vi "Overall_system_A1-125khz.vi"() -> ()   [LabVIEW 2019]
doc: "This VI is th overall VI that can read the weight, rfid and camera (and save the data into a csv file). When certain threshold are met it can also send a telegram message at the end."
uses:
  dependencies/notification/Telegram-Bot-master (1)/Telegram-Bot-master/Telegram/Methods/TypeDefs/SendMessageType.ctl
panel:
  out "Rfid":string
  in  "RFID VISA resource name 2":refnum<visa-resource-name>="COM1"
  in  "start condition (debug)":bool
  out "Weight":string
  in  "delay before read (ms)":u32=500
  in  "Weight VISA resource name":refnum<visa-resource-name>="COM1"
  in  "Start camera (debug)":bool
  out "Health Monitoring in Progress":bool
  in  "Bird is underfeeding (debug)":bool
  out "Current image":T1(plugin-control)
  in  "Camera Name":refnum<k21>="cam0" caption="IMAQdx Session"
  # "Intelligent Health Monitoring System"
  # "grams"
  # "Weight detection settings:"
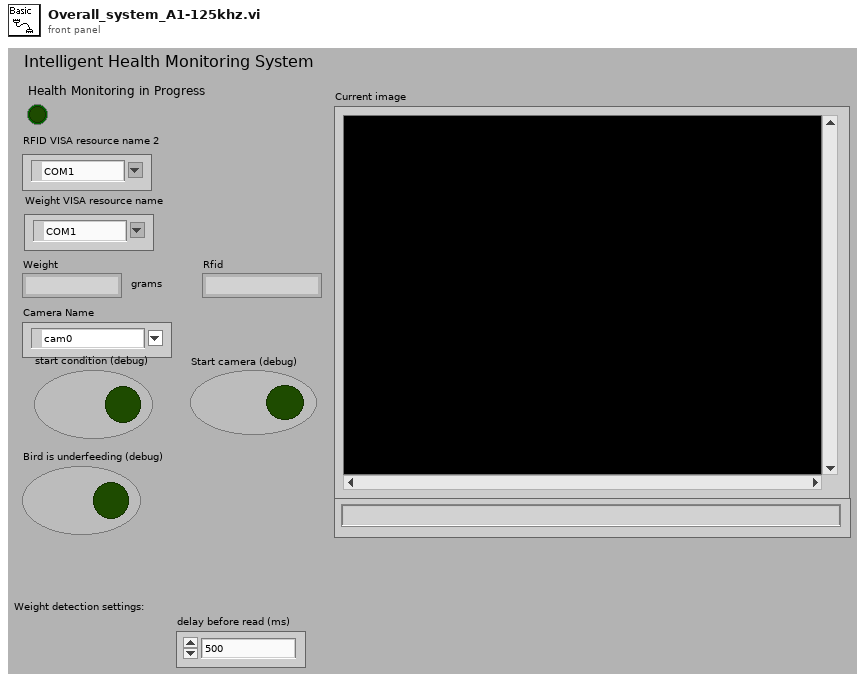
[diagram p1: front panel]
types:
  T1 = typedef "IMAQ Image.ctl" = refnum<image>
  T2 = typedef "SendMessageType.ctl" = enum16{"Text", "ReplyKeyboardMarkup", "ReplyKeyboardRemove"}
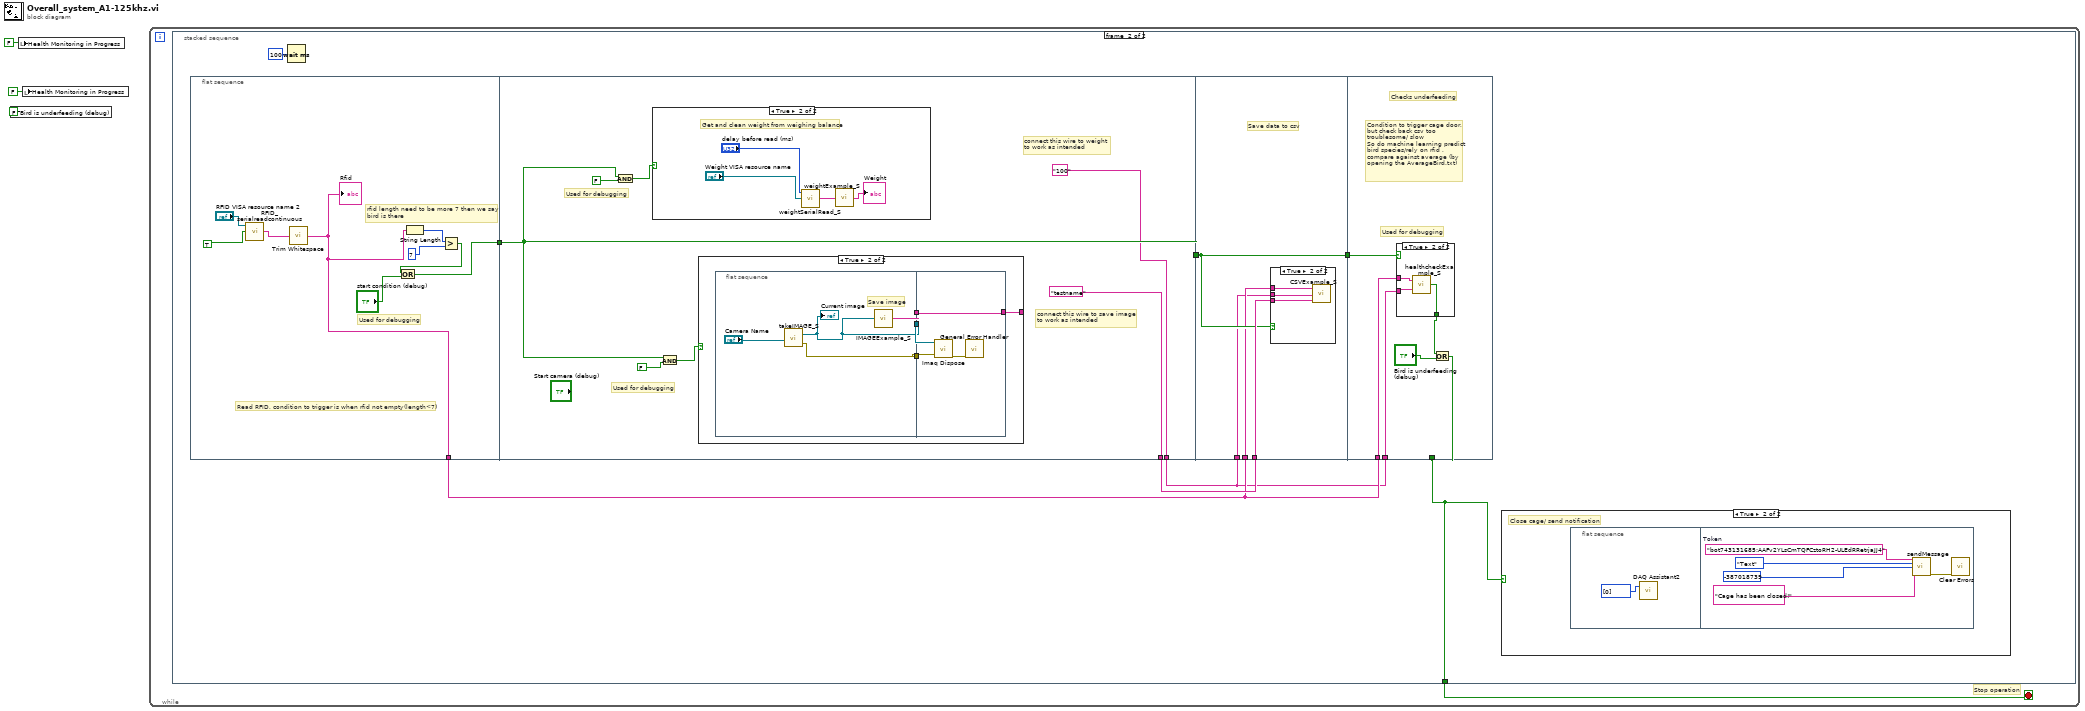
[diagram p0: block diagram]
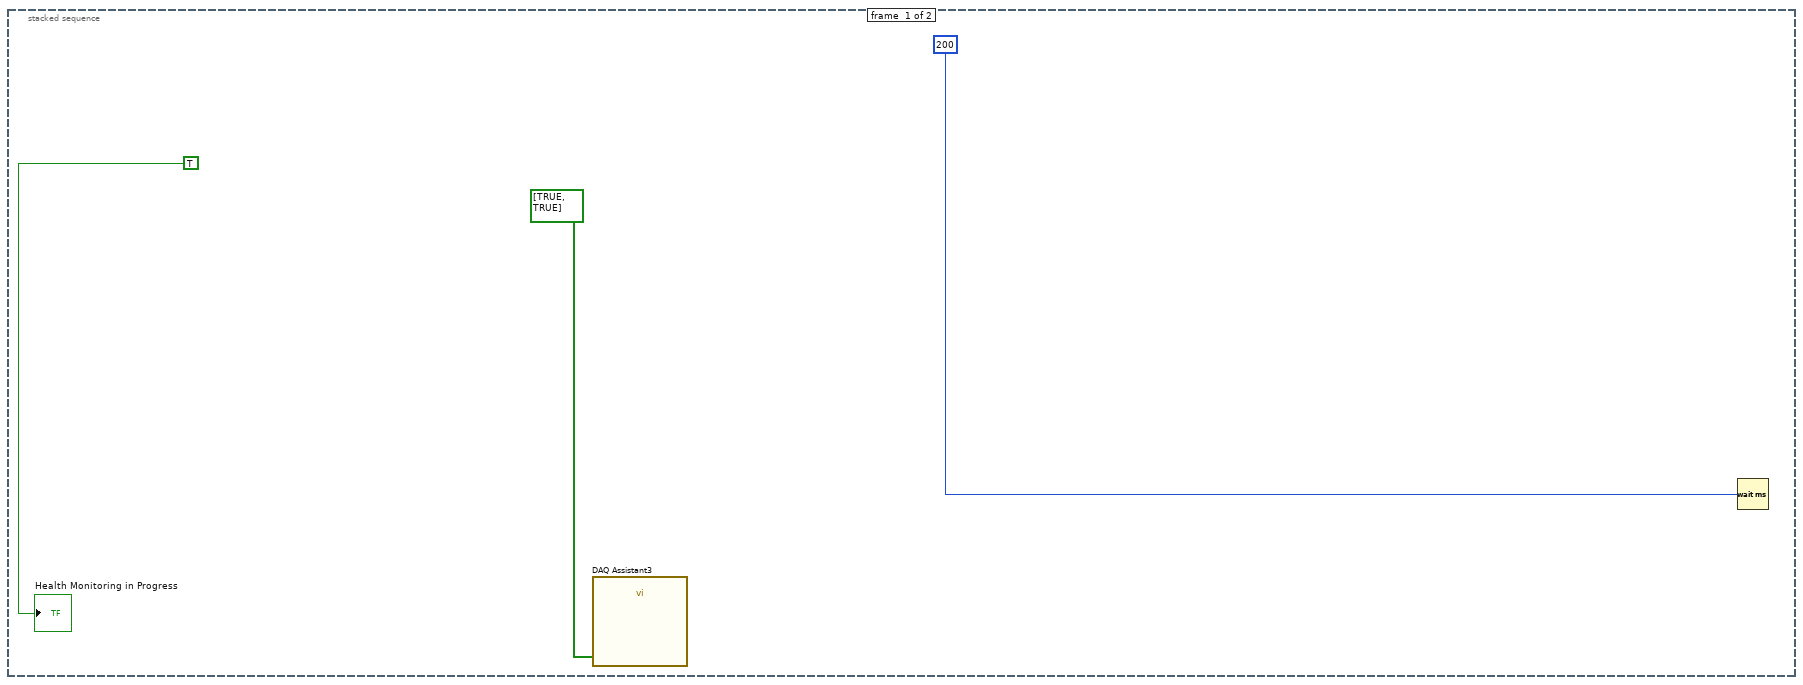
[diagram p2: hidden frame]
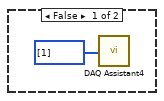
[diagram p4: hidden frame]
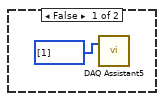
[diagram p7: hidden frame]
diagram:
  n1 = local write "Bird is underfeeding (debug)"(FALSE ("Bird is underfeeding")) -> ()
  n2 = local write "Health Monitoring in Progress"(FALSE ("Health Monitoring in Progress")) -> ()
  n3 = local write "Health Monitoring in Progress"(FALSE ("Health Monitoring in Progress")) -> ()
  n4 = while {
    stop <- w4 stop-if-true
    # "Stop operation"
    n5 = stacked-sequence {
      tunnel: [_ w14] -> w4
      frame #0 {
        n6 = call "DAQ Assistant3"("data"=bool[] [TRUE, TRUE]) -> ()  [unwired: 17 in, 2 out]
        n7 = Wait (ms)(milliseconds to wait=u32 200) -> ()  [unwired: 1 out]
        "Health Monitoring in Progress" <- TRUE ("Health Monitoring in Progress")
      }
      frame #1 {
        n8 = flat-sequence {
          tunnel: [w19] -> w9
          tunnel: [w23] -> w13
          tunnel: ["100"] -> w8
          tunnel: ["testname"] -> w10
          tunnel: w13 -> [w27]
          tunnel: [w27] -> w12
          tunnel: w12 -> [w51]
          tunnel: [w51] -> w11
          tunnel: w10 -> [w52]
          tunnel: w9 -> [w50]
          tunnel: w8 -> [w49]
          tunnel: [w58] -> w14
          tunnel: w9 -> [w57]
          tunnel: w11 -> [w61]
          tunnel: w8 -> [w56]
          frame #0 {
            # "Used for debugging"
            # "rfid length need to be more 7 then we say \nbird is there"
            # "Read RFID, condition to trigger is when rfid not empty(length<7)"
            n9 = call "RFID_serialreadcontinuous.vi"("Read 2"=TRUE, "VISA resource name"="RFID VISA resource name 2") -> ("Response 2"=w18:string)  [unwired: 1 in]
            n10 = call <vilib>:"Trim Whitespace.vi"("string"=w18) -> ("trimmed string"=w19:string)  [unwired: 1 in]
            "Rfid" <- w19
            n11 = String Length(string=w19) -> (length=w22:i32)
            n12 = Greater?(x=w22, y=7) -> (0:w20:bool)
            n13 = Or(x=w20, y="start condition (debug)") -> (x .or. y?=w23:bool)
          }
          frame #1 {
            # "connect this wire to save image \nto work as intended"
            # "connect this wire to weight \nto work as intended"
            # "Used for debugging"
            # "Used for debugging"
            n14 = And(x=w27, y=FALSE) -> (x .and. y?=w26:bool)
            n15 = case shown="True" w26 {
              frame False {
                n16 = call "DAQ Assistant4"("data"=u32[] [1]) -> ()  [unwired: 17 in, 2 out]
              }
              frame True {
                # "Get and clean weight from weighing balance"
                n17 = call "weightSerialRead_S.vi"("Weight VISA resource name"="Weight VISA resource name", "delay before read (ms)"="delay before read (ms)") -> ("String"=w48:string)  [unwired: 1 in]
                n18 = call "weightExample_S.vi"("weight"=w48) -> ("String"=→"Weight":string)
              }
            }
            n19 = And(x=w27, y=FALSE) -> (x .and. y?=w30:bool)
            n20 = case shown="True" w30 {
              tunnel: [_ w33] -> _
              frame False {
              }
              frame True {
                n21 = flat-sequence {
                  tunnel: [w37] -> w35
                  tunnel: [w36] -> w34
                  tunnel: [w39] -> w32
                  tunnel: w35 -> [w43]
                  tunnel: w34 -> [w41]
                  tunnel: [w40] -> w33
                  tunnel: w32 -> [w40]
                  frame #0 {
                    # "Save image"
                    n22 = call "takeIMAGE_S.vi"("Camera Name"="Camera Name") -> ("Current image"=w36:T1, "error in (no error)"=w37:errorcluster)
                    "Current image" <- w36
                    n23 = call "IMAGEExample_S.vi"("Image"=w36) -> ("String"=w39:string)
                  }
                  frame #1 {
                    n24 = call "Imaq Dispose"("Image"=w41, "error in (no error)"=w43) -> ("error out"=w42:errorcluster)  [unwired: 4 in]
                    n25 = call <vilib>:"General Error Handler.vi"("error in (no error)"=w42) -> ()  [unwired: 2 in, 13 out]
                  }
                }
              }
            }
          }
          frame #2 {
            # "Save data to csv"
            n26 = case shown="True" w51 {
              tunnel: w52 -> [_ w53]
              tunnel: w49 -> [_ w54]
              tunnel: w50 -> [_ w55]
              frame False {
              }
              frame True {
                n27 = call "CSVExample_S.vi"("imageId"=w53, "weight"=w54, "rfid"=w55) -> ()
              }
            }
          }
          frame #3 {
            # "Used for debugging"
            # "Condition to trigger cage door,\nbut check back csv too troublesome/ slow\nSo do machine learning predict bird species/rely on rfid , compare against average (by opening the AverageBird.txt)"
            # "Checks underfeeding"
            n28 = case shown="True" w61 {
              tunnel: [_ w62] -> w60
              tunnel: w57 -> [_ w63]
              tunnel: w56 -> [_ w64]
              frame False {
              }
              frame True {
                n29 = call "healthcheckExample_S.vi"("weight"=w64, "rfid"=w63) -> ("Boolean"=w62:bool)
              }
            }
            n30 = Or(x=w60, y="Bird is underfeeding (debug)") -> (x .or. y?=w58:bool)
          }
        }
        n31 = Wait (ms)(milliseconds to wait=u32 100) -> ()  [unwired: 1 out]
        n32 = case shown="True" w14 {
          frame False {
            n33 = call "DAQ Assistant5"("data"=u32[] [1]) -> ()  [unwired: 17 in, 2 out]
          }
          frame True {
            # "Close cage/ send notification"
            n34 = flat-sequence {
              frame #0 {
                n35 = call "DAQ Assistant2"("data"=u32[] [0]) -> ()  [unwired: 17 in, 2 out]
              }
              frame #1 {
                w70 = "bot743131685:AAFv2YLsCmTQFCztoRH2-ULEdRRetrjaJJ4"  # Token
                n36 = call "sendMessage.vi"("Token"=w70, "MsgType"=SendMessageType."Text", "ChatId"=i64 -387018739, "Text"="Cage has been closed!") -> ("error out"=w71:errorcluster)  [unwired: 11 in]
                n37 = call <vilib>:"Clear Errors.vi"("error in (no error)"=w71) -> ()  [unwired: 5 in, 2 out]
              }
            }
          }
        }
      }
    }
  }
